vi "isFriend.vi"(2 "error in (no error)":errorcluster, 3 "Friends":string[](array[string])) -> (0 "error out":errorcluster, 1 "isFriend?":bool)   [LabVIEW 2014, in "HGF_Auxiliary.lvlib"]
doc: "This VI can be used to check at runtime whether the caller-VI is a method of a friend class.\n\nThe owning class is automatically included."
uses:
  HGF_Auxiliary.lvlib
  ErrorCode.ctl
  Severity.ctl
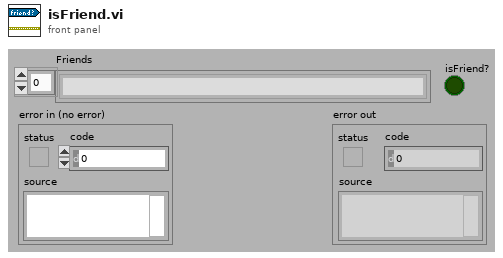
[diagram p1: front panel]
types:
  T1 = typedef "HGF_Auxiliary.lvlib/Severity.ctl" = enum16{"Info", "Warning", "Fault", "Error", "Fatal"}
  T2 = typedef "HGF_Auxiliary.lvlib/ErrorCode.ctl" = enum32{"No error", "Function not supported.", "This VI is for friends only.", "Reference object aready exisits.", "Parameter out of range.", "Not a rendezvous.", "Invalid notifier reference.", "Invalid queue reference.", "Self-Test not supported.", "Reset not supported.", "IDN query not supported.", "Error query not supported.", "Incorrect addressee.", "Object already exists.", "No class name specified", "Driver not supported", "Attribute is not writable"}
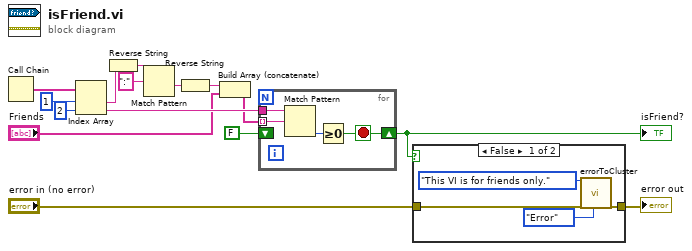
[diagram p0: block diagram]
diagram:
  n1 = Call Chain() -> (call chain=w14:string[])
  n2 = Index Array(array=w14, index #1=1 ("index"), index #2=2 ("index")) -> (element #1=w7:string, element #2=w13:string)
  n3 = Reverse String(1:w7) -> (0:w6:string)
  n4 = Match Pattern(string=w6, regular expression=":") -> (after substring=w4:string)  [unwired: 4 out]
  n5 = Reverse String(1:w4) -> (0:w3:string)
  n6 = Build Array (concatenate)(w3, "Friends") -> (w1:string[])
  n7 = for {
    tunnel: w13 -> [w19]
    shift-right: [w17] -> w9
    shift-left: FALSE -> [_]
    tunnel: w1 -> [w16] mode=indexing
    stop <- w17 stop-if-true
    n8 = Match Pattern(string=w19, regular expression=w16) -> (offset past match=w18:i32)  [unwired: 4 out]
    n9 = Greater Or Equal To 0?(x=w18) -> (x >= 0?=w17:bool)
  }
  "isFriend?" <- w9
  n10 = case shown="False" w9 {
    tunnel: "error in (no error)" -> [w22 w24]
    tunnel: [w23 w24] -> w10
    frame False {
      n11 = call "errorToCluster.vi"("error code"=ErrorCode."This VI is for friends only.", "error in (no error)"=w22, "severity (Error)"=Severity."Error") -> ("error out"=w23:errorcluster)  [unwired: 2 in, 14 out]
    }
    frame True {
    }
  }
  "error out" <- w10
